vi "Check valid stack ID.vi"(6 "Is real run?":bool, 8 "error in (no error)":errorcluster, 11 "Stack in":refnum<class "Stack.lvclass">) -> (0 "error out":errorcluster, 1 "Non-empty part IDs?":bool, 2 "Valid module ID?":bool, 3 "Stack out":refnum<class "Stack.lvclass">, 4 "Continue with current parts":bool, 5 "Non-empty assembly tray ID?":bool)   [LabVIEW 2021, in "Stack.lvclass"]
uses:
  Stack.lvclass
  Stack.lvclass/Stack.ctl
  Assembly/Database Entry/Database Entry.lvclass
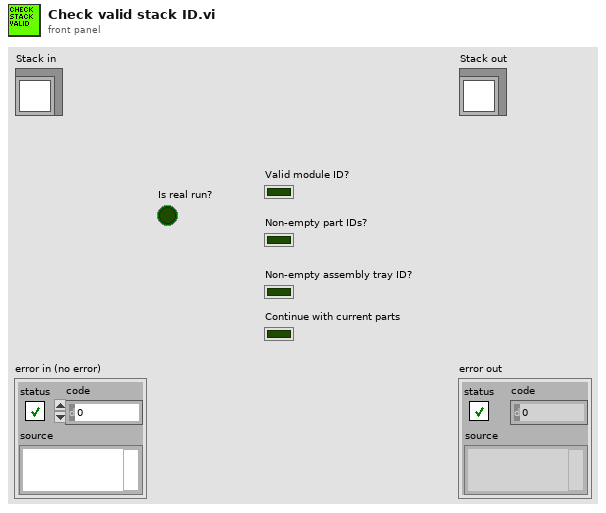
[diagram p1: front panel]
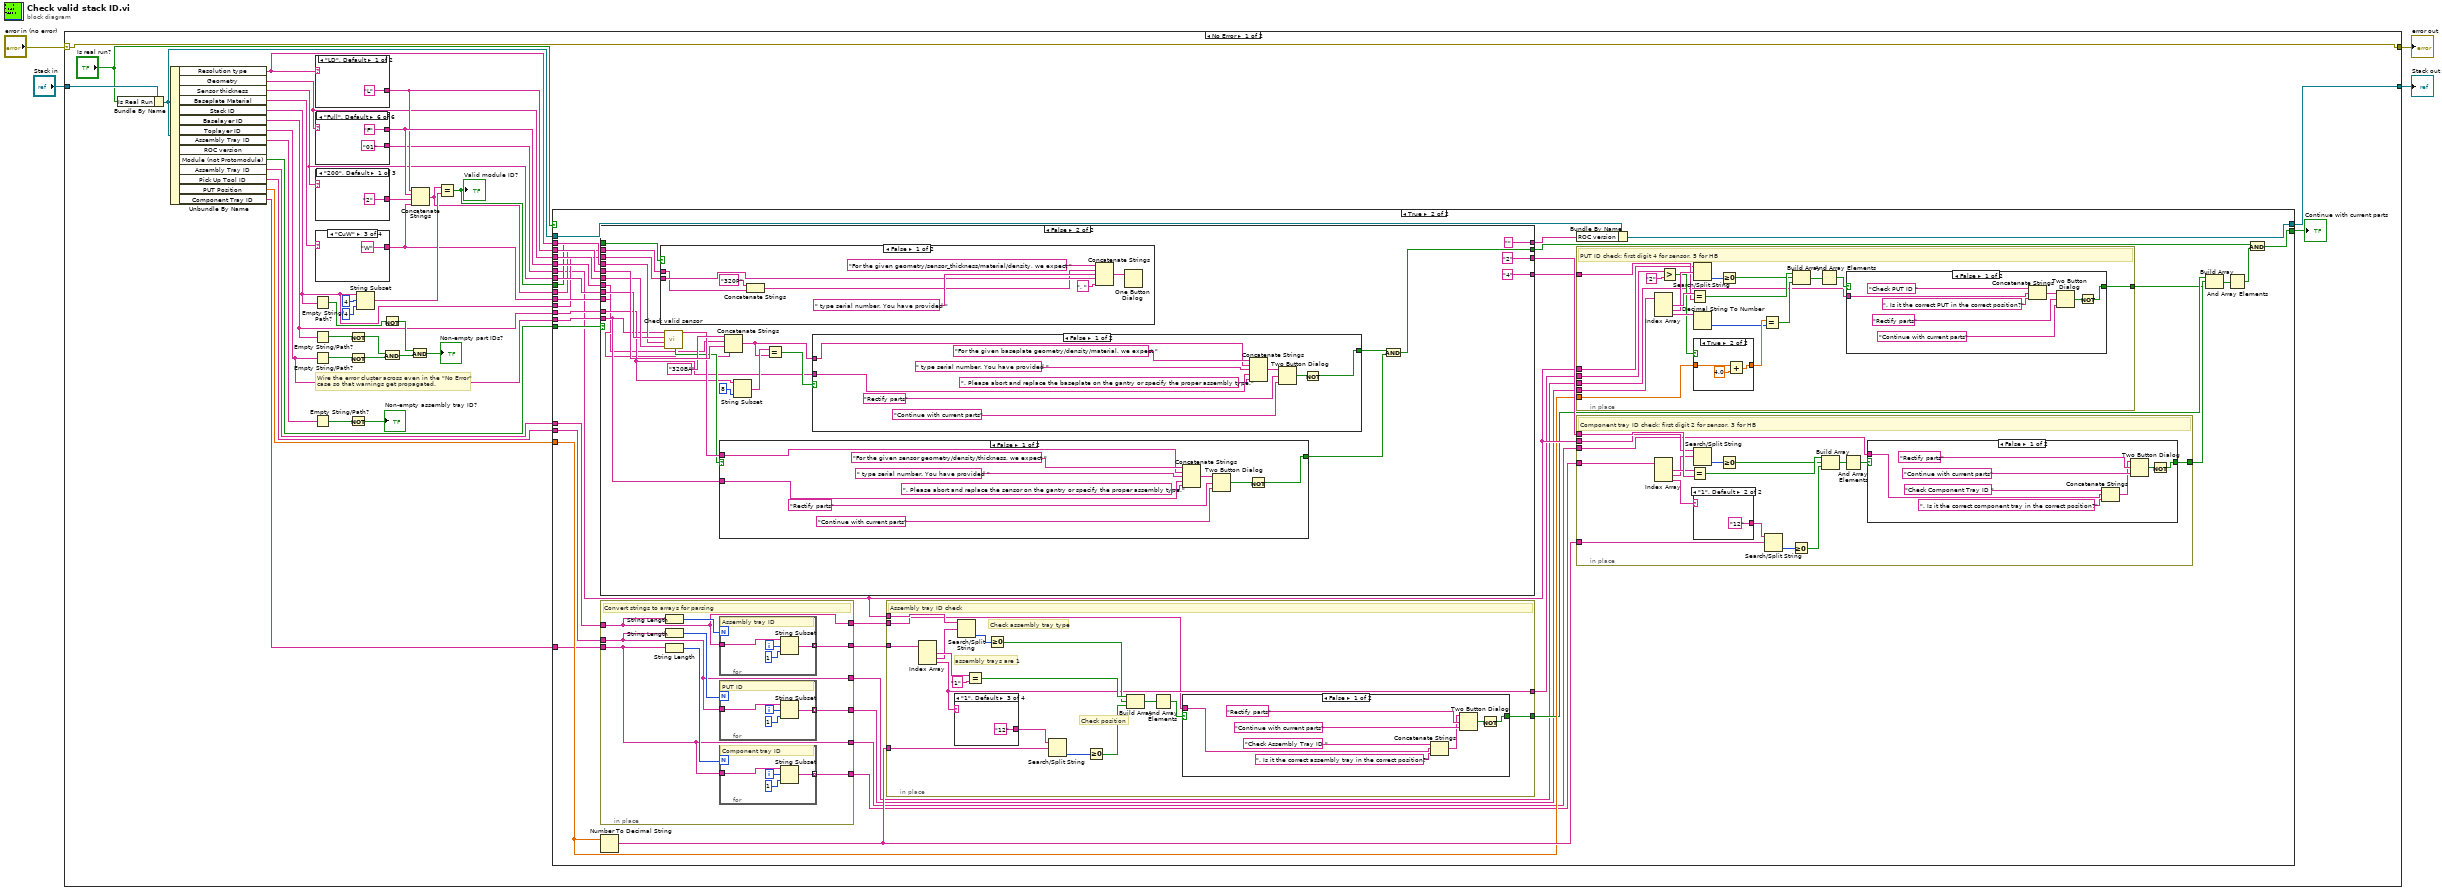
[diagram p0: block diagram]
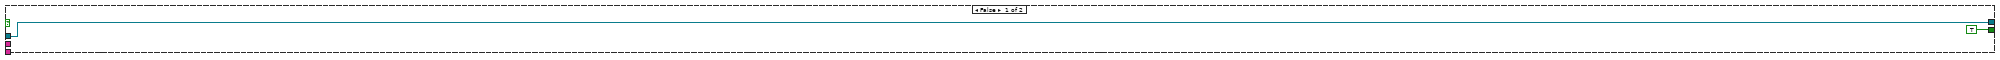
[diagram p2: hidden frame]
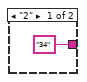
[diagram p5: hidden frame]
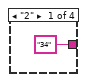
[diagram p7: hidden frame]
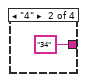
[diagram p8: hidden frame]
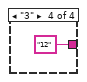
[diagram p9: hidden frame]
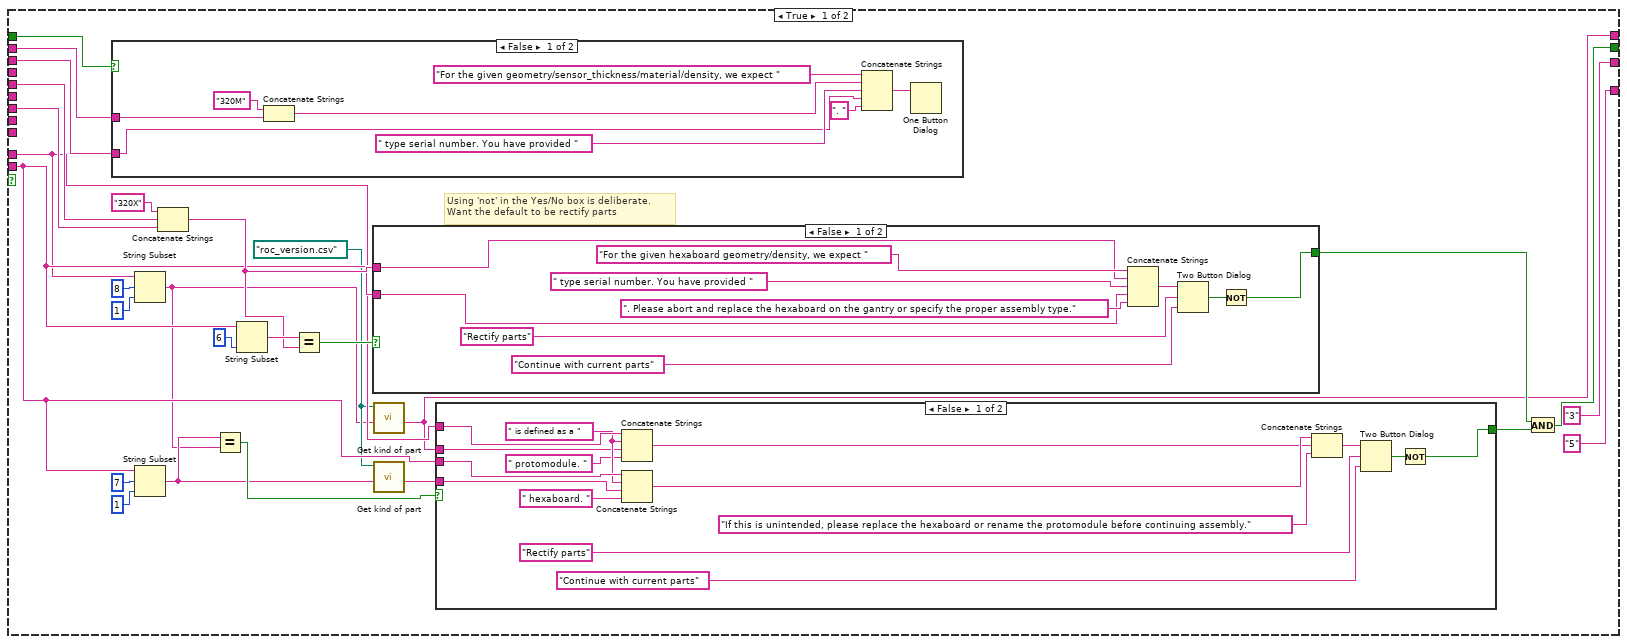
[diagram p11: hidden frame]
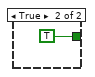
[diagram p13: hidden frame]
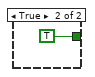
[diagram p14: hidden frame]
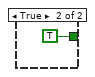
[diagram p16: hidden frame]
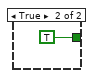
[diagram p17: hidden frame]
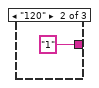
[diagram p18: hidden frame]
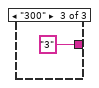
[diagram p19: hidden frame]
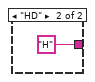
[diagram p20: hidden frame]
diagram:
  n1 = case shown="No Error" "error in (no error)" {
    selector: "error in (no error)" -> [w43 w333]
    tunnel: [w43 w333] -> w3
    tunnel: [w16 w332] -> w1
    tunnel: "Stack in" -> [w26 w332]
    frame No Error {
      # "Wire the error cluster across even in the \"No Error\"\ncase so that warnings get propagated."
      n2 = Bundle By Name(cluster=w26, "Is Real Run"="Is real run?") -> (w25:refnum<class "Stack.lvclass">)
      n3 = Unbundle By Name(w25) -> ("Resolution type"=w19:string, "Geometry"=w20:string, "Sensor thickness"=w17:string, "Baseplate Material"=w42:string, "Stack ID"=w14:string, "Baselayer ID"=w18:string, "Toplayer ID"=w21:string, "Assembly Tray ID"=w31:string, "Module (not Protomodule)"=w15:bool, "Assembly Tray ID"=w7:string, "Pick Up Tool ID"=w5:string, "PUT Position"=w8:dbl, "Component Tray ID"=w6:string)  [unwired: 1 out]
      n4 = Empty String/Path?(string/path=w14) -> (empty?=w30:bool)
      n5 = Empty String/Path?(string/path=w18) -> (empty?=w37:bool)
      n6 = Empty String/Path?(string/path=w21) -> (empty?=w36:bool)
      n7 = Empty String/Path?(string/path=w31) -> (empty?=w33:bool)
      n8 = case shown="\"LD\", Default" w19 {
        tunnel: ["L" "H"] -> w23
        frame "LD", Default {
        }
        frame "HD" {
        }
      }
      n9 = case shown="\"Full\", Default" w20 {
        tunnel: ["T" "B" "L" "R" "5" "F"] -> w24
        tunnel: ["45" "45" "3" "3" "02" "01"] -> w9
        frame "Top" {
        }
        frame "Bottom" {
        }
        frame "Left" {
        }
        frame "Right" {
        }
        frame "Five" {
        }
        frame "Full", Default {
        }
      }
      n10 = case shown="\"200\", Default" w17 {
        tunnel: ["2" "1" "3"] -> w41
        frame "200", Default {
        }
        frame "120" {
        }
        frame "300" {
        }
      }
      n11 = case shown="\"CuW\"" w42 {
        tunnel: ["P" "C" "W" "T"] -> w22
        frame "PCB" {
        }
        frame "CF", Default {
        }
        frame "CuW" {
        }
        frame "Ti" {
        }
      }
      n12 = Not(x=w37) -> (.not. x?=w34:bool)
      n13 = Not(x=w36) -> (.not. x?=w35:bool)
      n14 = Not(x=w33) -> (.not. x?=→"Non-empty assembly tray ID?":bool)
      n15 = String Subset(string=w14, offset (0)=4, length (rest)=4 ("length (rest)")) -> (substring=w38:string)
      n16 = Not(x=w30) -> (.not. x?=w29:bool)
      n17 = And(x=w34, y=w35) -> (x .and. y?=w28:bool)
      n18 = And(x=w29, y=w28) -> (x .and. y?=→"Non-empty part IDs?":bool)
      n19 = Concatenate Strings(w23, w24, w41, w22) -> (w13:string)
      n20 = Equal?(x=w13, y=w38) -> (x = y?=w12:bool)
      "Valid module ID?" <- w12
      n21 = case shown="True" "Is real run?" {
        tunnel: w25 -> [w44 w82]
        tunnel: w24 -> [_ w81]
        tunnel: w23 -> [_ w80]
        tunnel: w22 -> [_ w79]
        tunnel: w21 -> [_ w78]
        tunnel: w20 -> [_ w77]
        tunnel: w19 -> [_ w76]
        tunnel: w18 -> [_ w75]
        tunnel: w17 -> [_ w74]
        tunnel: [w44 w73] -> w16
        tunnel: w15 -> [_ w71]
        tunnel: w14 -> [_ w70]
        tunnel: w13 -> [_ w69]
        tunnel: w12 -> [_ w68]
        tunnel: [TRUE w66] -> w11
        tunnel: w9 -> [_ w62]
        tunnel: w8 -> [_ w61]
        tunnel: w7 -> [_ w54]
        tunnel: w6 -> [_ w53]
        tunnel: w5 -> [_ w52]
        frame False {
        }
        frame True {
          n22 = case shown="False" w71 {
            tunnel: w81 -> [w215 w261]
            tunnel: w80 -> [w216 w280]
            tunnel: w79 -> [_ w263]
            tunnel: w78 -> [w212 w268]
            tunnel: w77 -> [_ w274]
            tunnel: w74 -> [_ w273]
            tunnel: w76 -> [_ w272]
            tunnel: w75 -> [w211 w269]
            tunnel: [w205 w265] -> w67
            tunnel: [w200 "" ("String")] -> w72
            tunnel: w70 -> [w199 w262]
            tunnel: w69 -> [w197 w260]
            tunnel: w68 -> [w198 w259]
            tunnel: ["3" ("y") "2" ("y")] -> w65
            tunnel: ["5" ("y") "4" ("y")] -> w63
            frame True {
              w202 = path "roc_version.csv" ("name or relative path")
              # "Using 'not' in the Yes/No box is deliberate. \nWant the default to be rectify parts"
              n23 = case shown="False" w198 {
                tunnel: w199 -> [w225 _]
                tunnel: w197 -> [w224 _]
                frame False {
                  n24 = Concatenate Strings("320M" ("string"), w224) -> (w223:string)
                  n25 = Concatenate Strings("For the given geometry/sensor_thickness/material/density, we expect " ("message"), w223, " type serial number. You have provided " ("string"), w225, ". " ("string")) -> (w226:string)
                  n26 = One Button Dialog(message=w226) -> ()  [unwired: 1 in, 1 out]
                }
                frame True {
                }
              }
              n27 = String Subset(string=w211, offset (0)=8, length (rest)=1 ("length (rest)")) -> (substring=w201:string)
              n28 = String Subset(string=w212, offset (0)=7, length (rest)=1 ("length (rest)")) -> (substring=w204:string)
              n29 = Concatenate Strings("320X" ("string"), w216, w215) -> (w219:string)
              n30 = Equal?(x=w204, y=w201) -> (x = y?=w208:bool)
              n31 = String Subset(string=w212, length (rest)=6 ("length (rest)")) -> (substring=w220:string)  [unwired: 1 in]
              n32 = Equal?(x=w220, y=w219) -> (x = y?=w218:bool)
              n33 = case shown="False" w218 {
                tunnel: w219 -> [w254 _]
                tunnel: w212 -> [w250 _]
                tunnel: [w248 TRUE] -> w207
                frame False {
                  n34 = Concatenate Strings("For the given hexaboard geometry/density, we expect " ("message"), w254, " type serial number. You have provided " ("string"), w250, ". Please abort and replace the hexaboard on the gantry or specify the proper assembly type." ("string")) -> (w252:string)
                  n35 = Two Button Dialog(message=w252, 1:"Continue with current parts" ("T button name (\"OK\")"), 2:"Rectify parts" ("F button name (\"Cancel\")")) -> (T button?=w249:bool)
                  n36 = Not(x=w249) -> (.not. x?=w248:bool)
                }
                frame True {
                }
              }
              n37 = call "Get kind of part.vi"("Element"=w201, "File Path"=w202) -> ("Element definiton out"=w200:string)  [unwired: 9 in]
              n38 = call "Get kind of part.vi"("Element"=w204, "File Path"=w202) -> ("Element definiton out"=w203:string)  [unwired: 9 in]
              n39 = case shown="False" w208 {
                tunnel: w212 -> [w244 _]
                tunnel: w203 -> [w243 _]
                tunnel: w211 -> [w241 _]
                tunnel: w200 -> [w234 _]
                tunnel: [w233 TRUE] -> w206
                frame False {
                  w240 = " is defined as a " ("string")
                  n40 = Concatenate Strings(w241, w240, w234, " protomodule. " ("string")) -> (w237:string)
                  n41 = Concatenate Strings(w244, w240, w243, " hexaboard. " ("string")) -> (w238:string)
                  n42 = Concatenate Strings(w238, w237, "If this is unintended, please replace the hexaboard or rename the protomodule before continuing assembly." ("string")) -> (w235:string)
                  n43 = Two Button Dialog(message=w235, 1:"Continue with current parts" ("T button name (\"OK\")"), 2:"Rectify parts" ("F button name (\"Cancel\")")) -> (T button?=w232:bool)
                  n44 = Not(x=w232) -> (.not. x?=w233:bool)
                }
                frame True {
                }
              }
              n45 = And(x=w207, y=w206) -> (x .and. y?=w205:bool)
            }
            frame False {
              n46 = case shown="False" w259 {
                tunnel: w262 -> [w284 _]
                tunnel: w260 -> [w283 _]
                frame False {
                  n47 = Concatenate Strings("320P" ("string"), w283) -> (w282:string)
                  n48 = Concatenate Strings("For the given geometry/sensor_thickness/material/density, we expect " ("message"), w282, " type serial number. You have provided " ("string"), w284, ". " ("string")) -> (w285:string)
                  n49 = One Button Dialog(message=w285) -> ()  [unwired: 1 in, 1 out]
                }
                frame True {
                }
              }
              n50 = call "Check valid sensor.vi"("Geometry in"=w274, "Resolution in"=w272, "Thickness in"=w273, "Sensor ID"=w268) -> ("Sensor ID out"=w275:string, "Sensor ID okay"=w271:bool)  [unwired: 3 in, 3 out]
              n51 = case shown="False" w271 {
                tunnel: w275 -> [w297 _]
                tunnel: w268 -> [w293 _]
                tunnel: [w291 TRUE] -> w266
                frame False {
                  n52 = Concatenate Strings("For the given sensor geometry/density/thickness, we expect " ("message"), w297, " type serial number. You have provided " ("string"), w293, ". Please abort and replace the sensor on the gantry or specify the proper assembly type." ("string")) -> (w295:string)
                  n53 = Two Button Dialog(message=w295, 1:"Continue with current parts" ("T button name (\"OK\")"), 2:"Rectify parts" ("F button name (\"Cancel\")")) -> (T button?=w292:bool)
                  n54 = Not(x=w292) -> (.not. x?=w291:bool)
                }
                frame True {
                }
              }
              n55 = Concatenate Strings("320BA" ("string"), w261, w280, w263) -> (w276:string)
              n56 = String Subset(string=w269, length (rest)=8 ("length (rest)")) -> (substring=w277:string)  [unwired: 1 in]
              n57 = Equal?(x=w277, y=w276) -> (x = y?=w270:bool)
              n58 = case shown="False" w270 {
                tunnel: w276 -> [w308 _]
                tunnel: w269 -> [w304 _]
                tunnel: [w302 TRUE] -> w267
                frame False {
                  n59 = Concatenate Strings("For the given baseplate geometry/density/material, we expect " ("message"), w308, " type serial number. You have provided " ("string"), w304, ". Please abort and replace the baseplate on the gantry or specify the proper assembly type." ("string")) -> (w306:string)
                  n60 = Two Button Dialog(message=w306, 1:"Continue with current parts" ("T button name (\"OK\")"), 2:"Rectify parts" ("F button name (\"Cancel\")")) -> (T button?=w303:bool)
                  n61 = Not(x=w303) -> (.not. x?=w302:bool)
                }
                frame True {
                }
              }
              n62 = And(x=w267, y=w266) -> (x .and. y?=w265:bool)
            }
          }
          n63 = in-place {
            in-place-border: w54 -> [w83]
            in-place-border: [w90] -> w51
            in-place-border: w53 -> [w84]
            in-place-border: [w88] -> w50
            in-place-border: w52 -> [w85]
            in-place-border: [w86] -> w49
            in-place-border: [w85] -> w48
            in-place-border: [w84] -> w47
            in-place-border: [w83] -> w46
            # "Convert strings to arrays for parsing"
            n64 = String Length(string=w83) -> (length=w91:i32)
            n65 = String Length(string=w85) -> (length=w87:i32)
            n66 = String Length(string=w84) -> (length=w89:i32)
            n67 = for {
              N: w91 -> [_]
              tunnel: w83 -> [w103]
              tunnel: [w100] -> w90 mode=indexing
              i -> [w101]
              # "Assembly tray ID"
              n68 = String Subset(string=w103, offset (0)=w101, length (rest)=1 ("length (rest)")) -> (substring=w100:string)
            }
            n69 = for {
              N: w87 -> [_]
              tunnel: w85 -> [w95]
              tunnel: [w92] -> w86 mode=indexing
              i -> [w93]
              # "PUT ID"
              n70 = String Subset(string=w95, offset (0)=w93, length (rest)=1 ("length (rest)")) -> (substring=w92:string)
            }
            n71 = for {
              N: w89 -> [_]
              tunnel: w84 -> [w99]
              tunnel: [w96] -> w88 mode=indexing
              i -> [w97]
              # "Component tray ID"
              n72 = String Subset(string=w99, offset (0)=w97, length (rest)=1 ("length (rest)")) -> (substring=w96:string)
            }
          }
          n73 = Number To Decimal String(number=w61) -> (decimal integer string=w64:string)  [unwired: 1 in]
          n74 = in-place {
            in-place-border: w51 -> [w180]
            in-place-border: w62 -> [w168]
            in-place-border: [w176] -> w59
            in-place-border: w64 -> [w167]
            in-place-border: [w166] -> w60
            in-place-border: w46 -> [w165]
            # "Check position"
            # "Check assembly tray type"
            # "assembly trays are 1"
            # "Assembly tray ID check"
            n75 = Index Array(array=w180) -> (element #1=w179:string, element #2=w177:string, element #3=w166:string)  [unwired: 3 in]
            n76 = case shown="\"1\", Default" w166 {
              tunnel: ["34" ("string") "34" ("string") "12" ("string") "12" ("string")] -> w175
              frame "2" {
              }
              frame "4" {
              }
              frame "1", Default {
              }
              frame "3" {
              }
            }
            n77 = Search/Split String(string=w168, search string/char (-)=w177) -> (offset of match=w178:i32)  [unwired: 1 in, 2 out]
            n78 = Equal?(x=w179, y="1") -> (x = y?=w173:bool)
            n79 = Greater Or Equal To 0?(x=w178) -> (x >= 0?=w172:bool)
            n80 = Search/Split String(string=w175, search string/char (-)=w167) -> (offset of match=w174:i32)  [unwired: 1 in, 2 out]
            n81 = Greater Or Equal To 0?(x=w174) -> (x >= 0?=w171:bool)
            n82 = Build Array(w173, w172, w171) -> (w170:bool[])
            n83 = And Array Elements(Boolean array=w170) -> (logical AND=w169:bool)
            n84 = case shown="False" w169 {
              selector: w169 -> [_ w194]
              tunnel: [w190 w194] -> w176
              tunnel: w165 -> [w186 _]
              frame False {
                n85 = Concatenate Strings("Check Assembly Tray ID " ("string"), w186, ". Is it the correct assembly tray in the correct position?" ("string")) -> (w188:string)
                n86 = Two Button Dialog(message=w188, 1:"Continue with current parts" ("T button name (\"OK\")"), 2:"Rectify parts" ("F button name (\"Cancel\")")) -> (T button?=w191:bool)
                n87 = Not(x=w191) -> (.not. x?=w190:bool)
              }
              frame True {
              }
            }
          }
          n88 = Bundle By Name(cluster=w82, "ROC version"=w72) -> (w73:refnum<class "Stack.lvclass">)
          n89 = in-place {
            in-place-border: w49 -> [w123]
            in-place-border: [w121] -> w57
            in-place-border: w63 -> [w114]
            in-place-border: w62 -> [w113]
            in-place-border: w61 -> [w108]
            in-place-border: w60 -> [w110]
            in-place-border: w48 -> [w104]
            # "PUT ID check: first digit 4 for sensor, 5 for HB"
            n90 = Index Array(array=w123) -> (element #1=w122:string, element #2=w120:string, element #3=w112:string)  [unwired: 3 in]
            n91 = Greater?(x=w110, y="2") -> (0:w111:bool)
            n92 = Equal?(x=w122, y=w114) -> (x = y?=w118:bool)
            n93 = Search/Split String(string=w113, search string/char (-)=w120) -> (offset of match=w119:i32)  [unwired: 1 in, 2 out]
            n94 = Decimal String To Number(string=w112) -> (number=w106:i32)  [unwired: 2 in, 1 out]
            n95 = case shown="True" w111 {
              tunnel: w108 -> [w124 w127]
              tunnel: [w124 w125] -> w107
              frame False {
              }
              frame True {
                n96 = Add(x=w127, y=4.0) -> (x+y=w125:dbl)
              }
            }
            n97 = Greater Or Equal To 0?(x=w119) -> (x >= 0?=w117:bool)
            n98 = Equal?(x=w107, y=w106) -> (x = y?=w105:bool)
            n99 = Build Array(w118, w117, w105) -> (w116:bool[])
            n100 = And Array Elements(Boolean array=w116) -> (logical AND=w115:bool)
            n101 = case shown="False" w115 {
              selector: w115 -> [_ w136]
              tunnel: [w132 w136] -> w121
              tunnel: w104 -> [w130 _]
              frame False {
                n102 = Concatenate Strings("Check PUT ID " ("string"), w130, ". Is it the correct PUT in the correct position?" ("string")) -> (w128:string)
                n103 = Two Button Dialog(message=w128, 1:"Continue with current parts" ("T button name (\"OK\")"), 2:"Rectify parts" ("F button name (\"Cancel\")")) -> (T button?=w133:bool)
                n104 = Not(x=w133) -> (.not. x?=w132:bool)
              }
              frame True {
              }
            }
          }
          n105 = in-place {
            in-place-border: w50 -> [w153]
            in-place-border: w65 -> [w152]
            in-place-border: [w150] -> w58
            in-place-border: w62 -> [w149]
            in-place-border: w64 -> [w138]
            in-place-border: w47 -> [w137]
            # "Component tray ID check: first digit 2 for sensor, 3 for HB"
            n106 = Index Array(array=w153) -> (element #1=w151:string, element #2=w148:string, element #3=w140:string)  [unwired: 3 in]
            n107 = Equal?(x=w151, y=w152) -> (x = y?=w146:bool)
            n108 = Search/Split String(string=w149, search string/char (-)=w148) -> (offset of match=w147:i32)  [unwired: 1 in, 2 out]
            n109 = case shown="\"1\", Default" w140 {
              tunnel: ["34" ("string") "12" ("string")] -> w142
              frame "2" {
              }
              frame "1", Default {
              }
            }
            n110 = Greater Or Equal To 0?(x=w147) -> (x >= 0?=w145:bool)
            n111 = Search/Split String(string=w142, search string/char (-)=w138) -> (offset of match=w141:i32)  [unwired: 1 in, 2 out]
            n112 = Greater Or Equal To 0?(x=w141) -> (x >= 0?=w139:bool)
            n113 = Build Array(w146, w145, w139) -> (w144:bool[])
            n114 = And Array Elements(Boolean array=w144) -> (logical AND=w143:bool)
            n115 = case shown="False" w143 {
              selector: w143 -> [_ w164]
              tunnel: [w160 w164] -> w150
              tunnel: w137 -> [w158 _]
              frame False {
                n116 = Concatenate Strings("Check Component Tray ID " ("string"), w158, ". Is it the correct component tray in the correct position?" ("string")) -> (w157:string)
                n117 = Two Button Dialog(message=w157, 1:"Continue with current parts" ("T button name (\"OK\")"), 2:"Rectify parts" ("F button name (\"Cancel\")")) -> (T button?=w161:bool)
                n118 = Not(x=w161) -> (.not. x?=w160:bool)
              }
              frame True {
              }
            }
          }
          n119 = Build Array(w59, w58, w57) -> (w56:bool[])
          n120 = And Array Elements(Boolean array=w56) -> (logical AND=w55:bool)
          n121 = And(x=w67, y=w55) -> (x .and. y?=w66:bool)
        }
      }
      "Continue with current parts" <- w11
    }
    frame Error {
    }
  }
  "error out" <- w3
  "Stack out" <- w1
